vi "Get DAQChannel Info.vi"(8 "error in (no error)":errorcluster, 11 "Sequencer in":refnum<class "Sequencer.lvclass">) -> (0 "error out":errorcluster, 3 "Sequencer out":refnum<class "Sequencer.lvclass">)   [LabVIEW 2015, in "Sequencer.lvlib" / "Sequencer.lvclass"]
uses:
  Sequencer.lvclass
  Sequencer.lvclass/Sequencer.ctl
  <resource>/objmgr/daqmx.rc
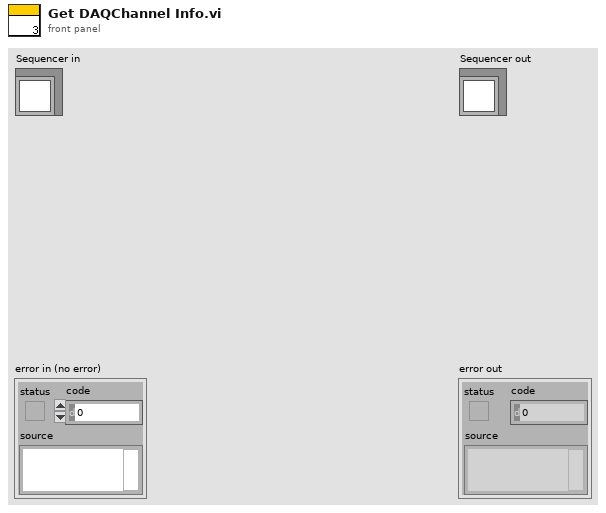
[diagram p1: front panel]
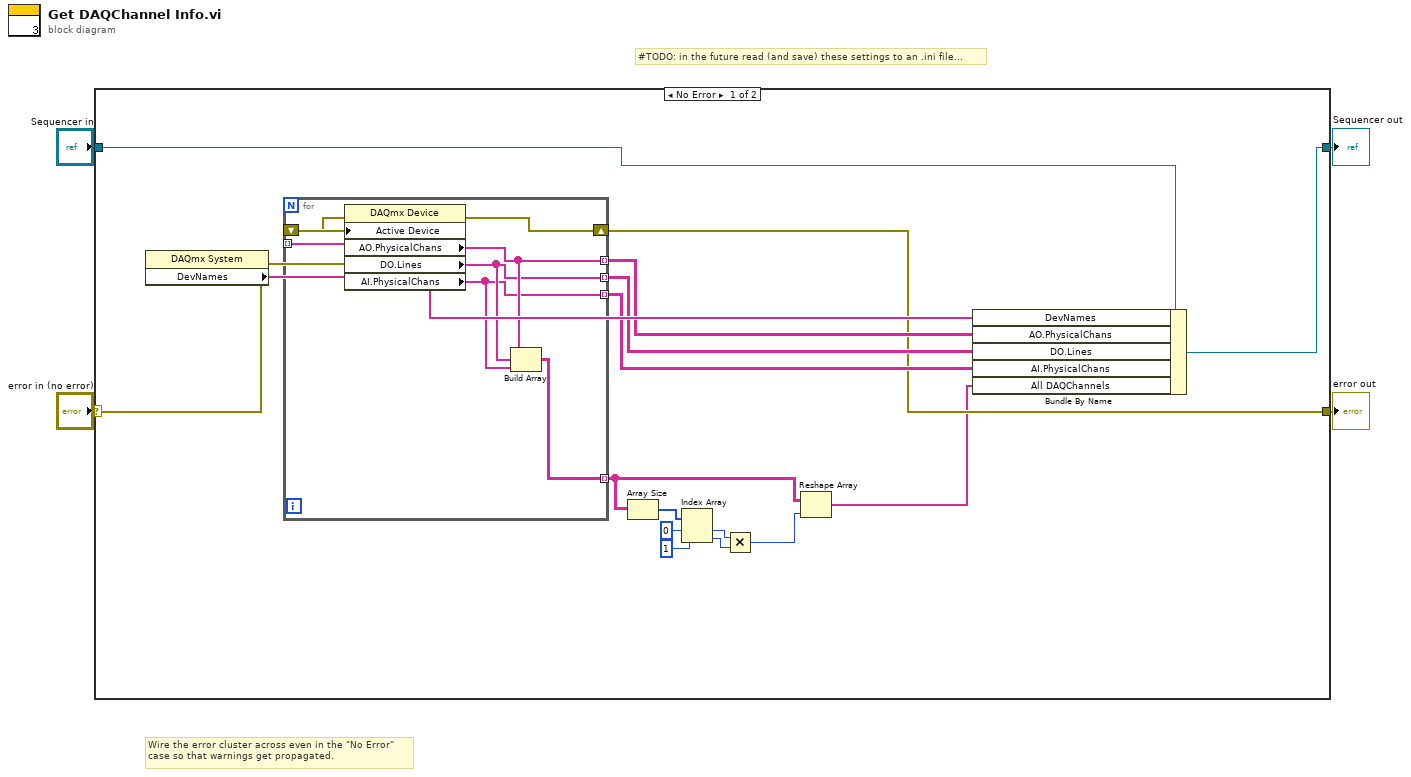
[diagram p0: block diagram]
diagram:
  # "Wire the error cluster across even in the \"No Error\"\ncase so that warnings get propagated."
  # "#TODO: in the future read (and save) these settings to an .ini file..."
  n1 = case shown="No Error" "error in (no error)" {
    selector: "error in (no error)" -> [w15 w30]
    tunnel: [w14 w30] -> w3
    tunnel: [w13 w29] -> w1
    tunnel: "Sequencer in" -> [w16 w29]
    frame No Error {
      n2 = property class="DAQmx System"(error in=w15) -> (error out=w21:errorcluster, "DevNames"=w20:tag[])  [unwired: 1 in, 1 out]
      n3 = for {
        tunnel: w20 -> [w28] mode=indexing
        tunnel: [w25] -> w17 mode=indexing
        tunnel: [w24] -> w18 mode=indexing
        tunnel: [w23] -> w19 mode=indexing
        shift-right: [w26] -> w14
        shift-left: w21 -> [w27]
        tunnel: [w22] -> w7 mode=indexing
        n4 = property class="DAQmx Device"(error in=w27, "Active Device"=w28) -> (error out=w26:errorcluster, "AO.PhysicalChans"=w25:tag[], "DO.Lines"=w24:tag[], "AI.PhysicalChans"=w23:tag[])  [unwired: 1 in, 1 out]
        n5 = Build Array(w25, w24, w23) -> (w22:tag[][])
      }
      n6 = Array Size(array=w7) -> (size(s)=w12:i32[])
      n7 = Index Array(array=w12, index #1=0 ("index"), index #2=1 ("index")) -> (element #1=w9:i32, element #2=w8:i32)
      n8 = Multiply(x=w9, y=w8) -> (x*y=w6:i32)
      n9 = Reshape Array(w7, w6) -> (w5:tag[])
      n10 = Bundle By Name(cluster=w16, "DevNames"=w20, "AO.PhysicalChans"=w17, "DO.Lines"=w18, "AI.PhysicalChans"=w19, "All DAQChannels"=w5) -> (w13:refnum<class "Sequencer.lvclass">)
    }
    frame Error {
    }
  }
  "error out" <- w3
  "Sequencer out" <- w1
